vi "checkpoint action 1.vi"(10 "Drone":T1) -> (2 "Drone":T1)   [LabVIEW 2009]
uses:
  Drone data.ctl
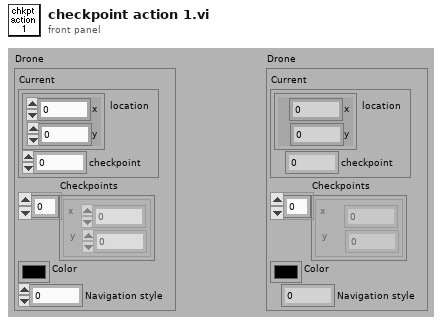
[diagram p1: front panel]
types:
  T1 = typedef "Drone data.ctl" = cluster{"Current":cluster{"location":cluster{"x":i16, "y":i16}, "checkpoint":i32}, "Checkpoints":cluster{"x":i16, "y":i16}[], "Color":u32, "Navigation style":i32}
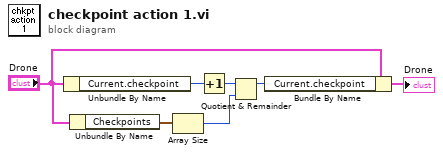
[diagram p0: block diagram]
diagram:
  n1 = Unbundle By Name("Drone") -> ("Current.checkpoint"=w5:i32)
  n2 = Unbundle By Name("Drone") -> ("Checkpoints"=w4:cluster{"x":i16, "y":i16}[])
  n3 = Array Size(array=w4) -> (size(s)=w1:i32)
  n4 = Increment(x=w5) -> (x+1=w3:i32)
  n5 = Quotient & Remainder(x=w3, y=w1) -> (x-y*floor(x/y)=w2:i32)  [unwired: 1 out]
  n6 = Bundle By Name(cluster="Drone", "Current.checkpoint"=w2) -> (→"Drone":T1)
